vi "dut_tx_test.vi"(11 "TV Parameters(DataType)":T1 {"Standard" items=["80211A/G/J/P OFDM", "80211B/G DSSS", "80211G DSSSOFDM", "80211N MIMOOFDM", "80211AC MIMOOFDM"]; "OFDM Data Rate (Mbps)" items=["6", "9", "12", "18", "24", "36", "48", "54"]; "80211n PLCP Frame Format" items=["Mixed Format", "Greenfield Format"]; "FEC Coding Type" items=["BCC", "LDPC"]; "DSSS Data Rate (Mbps)" items=["1", "2", "5.5 CCK", "5.5 PBCC", "11 CCK", "11 PBCC", "22", "33"]}) -> (3 "Command Sent":string)   [LabVIEW 2011]
uses:
  TV/RW/Includes/WLAN - TV - RW - INC - TV_DataType_Cluster.ctl
  Controls/Transmit Config.ctl
  Controls/Data Rates.ctl
  Controls/Inter Frame Spacing modes.ctl
  Controls/Parameter.ctl
panel:
  in  "OFDM Data Rate (Mbps)":i32(ring) items=["6", "9", "12", "18", "24", "36", "48", "54"]
  out "Messages Logged":string[](array[string])
  in  "error in (no error)":errorcluster
  out "error out":errorcluster
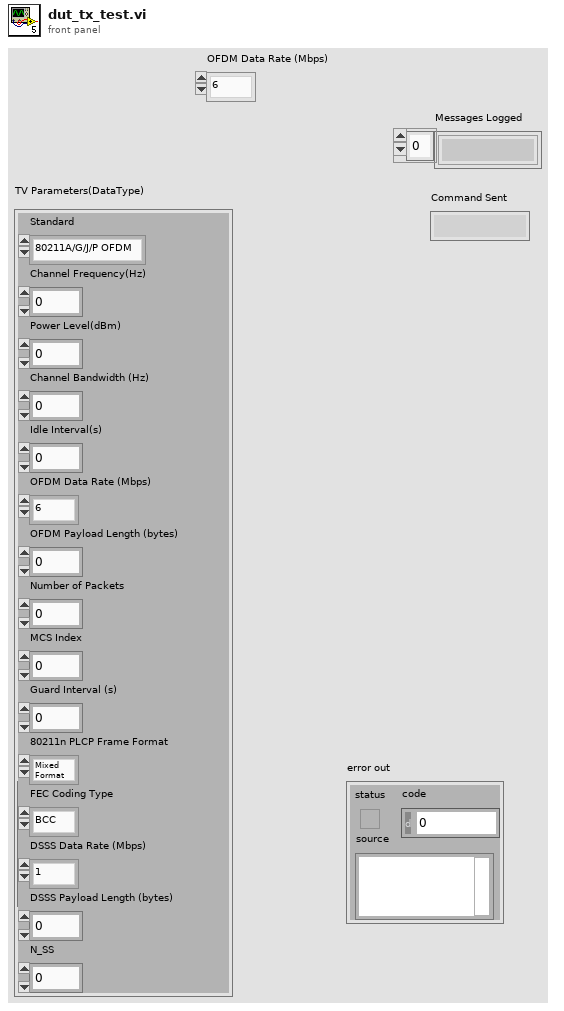
[diagram p1: front panel]
types:
  T1 = typedef "WLAN - TV - RW - INC - TV_DataType_Cluster.ctl" = cluster{"Standard":i32, "Channel Frequency(Hz)":dbl, "Power Level(dBm)":dbl, "Channel Bandwidth (Hz)":dbl, "Idle Interval(s)":dbl, "OFDM Data Rate (Mbps)":i32, "OFDM Payload Length (bytes)":i32, "Number of Packets":i32, "MCS Index":i32, "Guard Interval (s)":dbl, "80211n PLCP Frame Format":i32, "FEC Coding Type":i32, "DSSS Data Rate (Mbps)":i32, "DSSS Payload Length (bytes)":i32, "N_SS":i32}
  T2 = typedef "Data Rates.ctl" = string
  T3 = typedef "Transmit Config.ctl" = cluster{"Packet Length":u32, "Packet Count":i32, "Data Rate":T2, "Frequency, MHz":u32, "Continuous Frames":bool, "TX Power, dB":dbl}
  T4 = enum16{"none", "combined", "isolated", "iterate-combined ", "iterate-isolated"}
  T5 = typedef "Parameter.ctl" = cluster{"Name":string, "Type":enum16{"decimal", "string", "float", "hex"}}
  T6 = typedef "Inter Frame Spacing modes.ctl" = i16
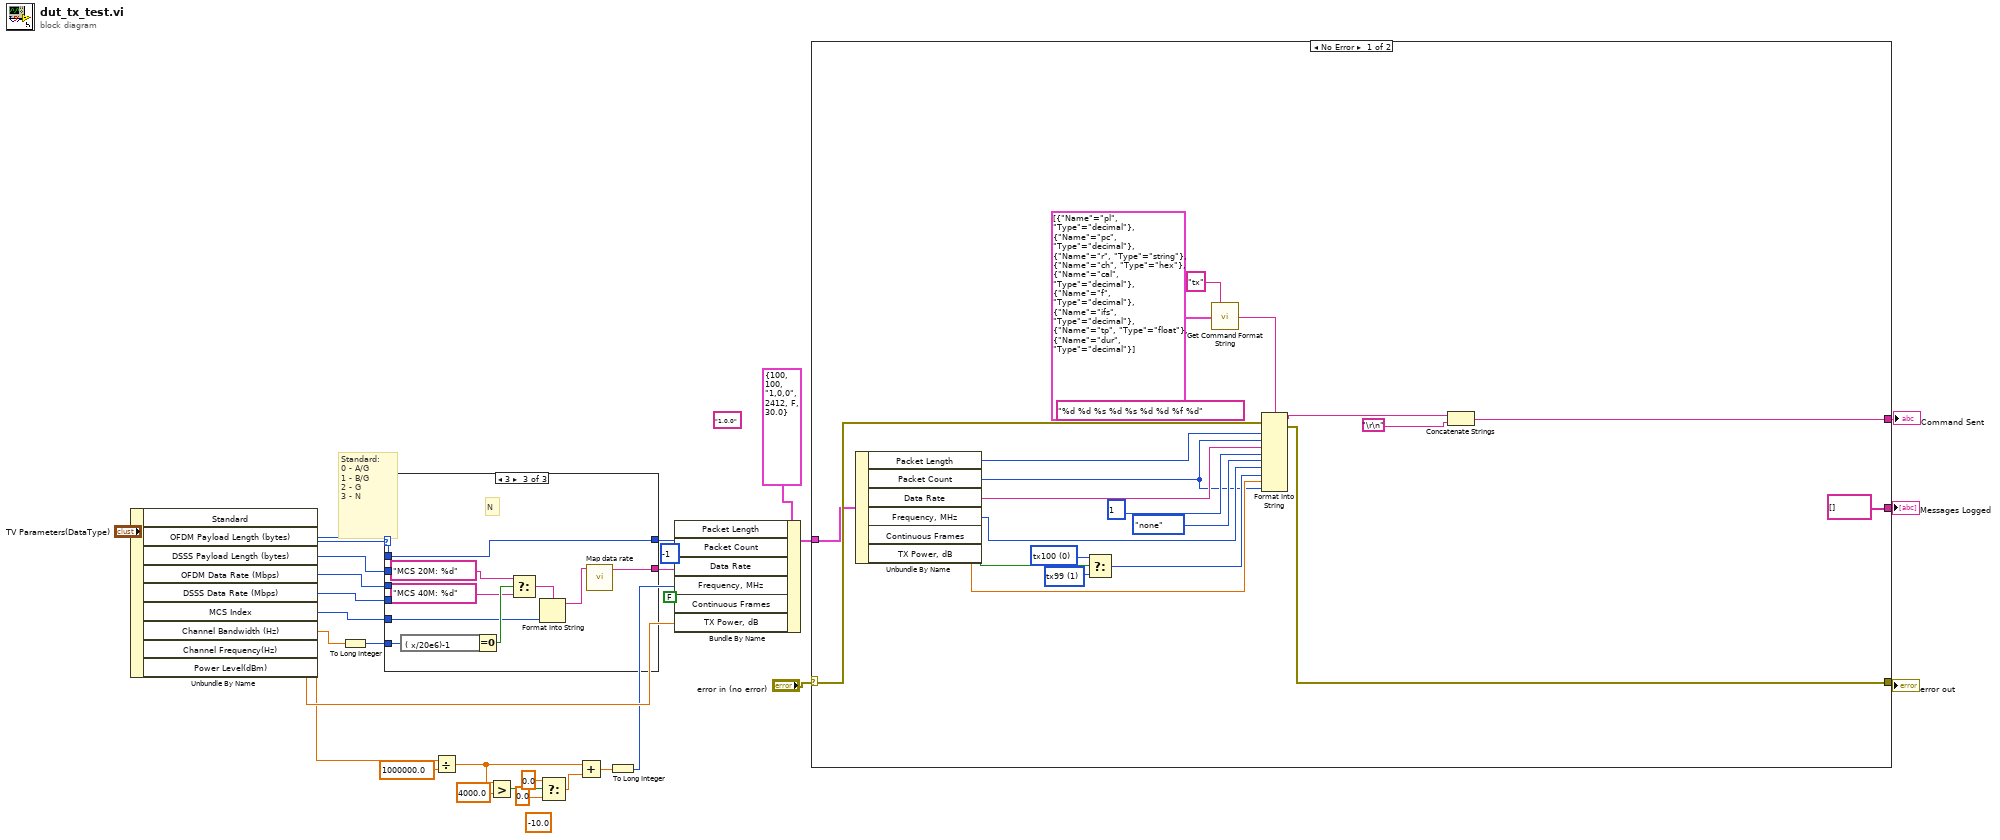
[diagram p0: block diagram]
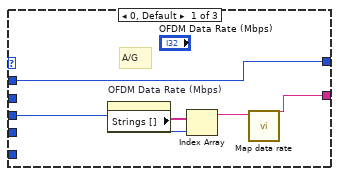
[diagram p2: hidden frame]
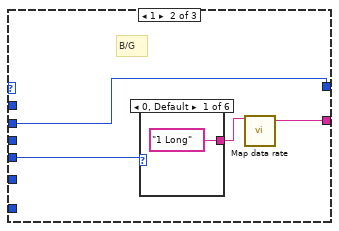
[diagram p3: hidden frame]
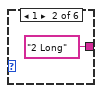
[diagram p4: hidden frame]
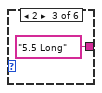
[diagram p5: hidden frame]
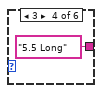
[diagram p6: hidden frame]
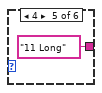
[diagram p7: hidden frame]
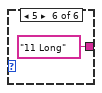
[diagram p8: hidden frame]
diagram:
  (unwired) -10.0 ("t")
  (unwired) T2 "1,0,0" ("Data Rate")
  # "Standard:\n0 - A/G\n1 - B/G\n2 - G\n3 - N"
  n1 = Unbundle By Name("TV Parameters(DataType)") -> ("Standard"=w21:i32, "OFDM Payload Length (bytes)"=w19:i32, "DSSS Payload Length (bytes)"=w18:i32, "OFDM Data Rate (Mbps)"=w17:i32, "DSSS Data Rate (Mbps)"=w15:i32, "MCS Index"=w14:i32, "Channel Bandwidth (Hz)"=w10:dbl, "Channel Frequency(Hz)"=w12:dbl, "Power Level(dBm)"=w16:dbl)
  n2 = To Long Integer(number=w10) -> (32bit integer=w9:i32)
  n3 = case shown="3" w21 {
    tunnel: [w35 w39 w55] -> w20
    tunnel: w19 -> [w35 _ w55]
    tunnel: w18 -> [_ w39 _]
    tunnel: w17 -> [w31 _ _]
    tunnel: w15 -> [_ w38 _]
    tunnel: w14 -> [_ _ w46]
    tunnel: [w34 w37 w54] -> w13
    tunnel: w9 -> [_ _ w47]
    frame 0, Default {
      # "A/G"
      n4 = property on="OFDM Data Rate (Mbps)" class="Ring (strict)"() -> ("Strings []"=w33:string[])  [unwired: 2 in, 2 out]
      n5 = Index Array(array=w33, index=w31) -> (element=w32:string)
      n6 = call "Map data rate.vi"("Data Rate In"=w32) -> ("Data Rate Out"=w34:string)  [unwired: 10 in]
    }
    frame 1 {
      # "B/G"
      n7 = case shown="0, Default" w38 {
        tunnel: ["1 Long" ("Data Rate In") "2 Long" ("Data Rate In") "5.5 Long" ("Data Rate In") "5.5 Long" ("Data Rate In") "11 Long" ("Data Rate In") "11 Long" ("Data Rate In")] -> w36
        frame 0, Default {
        }
        frame 1 {
        }
        frame 2 {
        }
        frame 3 {
        }
        frame 4 {
        }
        frame 5 {
        }
      }
      n8 = call "Map data rate.vi"("Data Rate In"=w36) -> ("Data Rate Out"=w37:string)  [unwired: 10 in]
    }
    frame 3 {
      # "N"
      n9 = expression code="( x/20e6)-1"(w47) -> (w51:i32)
      n10 = Equal To 0?(x=w51) -> (x = 0?=w52:bool)
      n11 = Select(t="MCS 20M: %d" ("format string"), s=w52, f="MCS 40M: %d" ("format string")) -> (s? t:f=w53:string)
      n12 = Format Into String(format string=w53, w46) -> (resulting string=w48:string)  [unwired: 2 in, 1 out]
      n13 = call "Map data rate.vi"("Data Rate In"=w48) -> ("Data Rate Out"=w54:string)  [unwired: 10 in]
    }
  }
  n14 = Divide(x=w12, y=1000000.0 ("x")) -> (x/y=w8:dbl)
  n15 = Greater?(x=w8, y=4000.0) -> (0:w6:bool)
  n16 = Select(t=0.0, s=w6, f=0.0) -> (s? t:f=w2:dbl)
  n17 = Add(x=w8, y=w2) -> (x+y=w3:dbl)
  n18 = To Long Integer(number=w3) -> (32bit integer=w1:i32)
  n19 = Bundle By Name(cluster=T3 {"Packet Length"=100, "Packet Count"=100, "Data Rate"="1,0,0", "Frequency, MHz"=2412, "Continuous Frames"=FALSE, "TX Power, dB"=30.0} ("Transmit Config"), "Packet Length"=w20, "Packet Count"=-1, "Data Rate"=w13, "Frequency, MHz"=w1, "Continuous Frames"=FALSE, "TX Power, dB"=w16) -> (w25:T3)
  n20 = case shown="No Error" "error in (no error)" {
    selector: "error in (no error)" -> [w76 w77]
    tunnel: [w56 w77] -> w29
    tunnel: [string[] [] ("Messages Logged") _] -> w28
    tunnel: [w69 _] -> w27
    tunnel: w25 -> [w57 _]
    frame No Error {
      (unwired) "%d %d %s %d %s %d %d %f %d" ("format string")
      w63 = T6 1 items=["Regular"=-1, "tx100"=0, "tx99"=1] ("ART2 Data.Transmit Config.Inter Frame Spacing")
      w64 = T6 0 items=["Regular"=-1, "tx100"=0, "tx99"=1] ("ART2 Data.Transmit Config.Inter Frame Spacing")
      n21 = Unbundle By Name(w57) -> ("Packet Length"=w75:u32, "Packet Count"=w60:i32, "Data Rate"=w67:T2, "Frequency, MHz"=w72:u32, "Continuous Frames"=w62:bool, "TX Power, dB"=w70:dbl)
      n22 = Select(t=w64, s=w62, f=w63) -> (s? t:f=w61:T6)
      n23 = call "Get Command Format String.vi"("Command"="tx", "Parameters"=T5[] [{"Name"="pl", "Type"=enum."decimal"}, {"Name"="pc", "Type"=enum."decimal"}, {"Name"="r", "Type"=enum."string"}, {"Name"="ch", "Type"=enum."hex"}, {"Name"="cal", "Type"=enum."decimal"}, {"Name"="f", "Type"=enum."decimal"}, {"Name"="ifs", "Type"=enum."decimal"}, {"Name"="tp", "Type"=enum."float"}, {"Name"="dur", "Type"=enum."decimal"}]) -> ("Command Format String"=w71:string)  [unwired: 13 in]
      n24 = Format Into String(format string=w71, error in=w76, w75, w60, w67, u32 1 ("Chains"), T4."none" ("input 5"), w72, w61, w70, w60) -> (resulting string=w59:string, error out=w56:errorcluster)  [unwired: 1 in]
      n25 = Concatenate Strings(w59, "\r\n") -> (w69:string)
    }
    frame Error {
    }
  }
  "error out" <- w29
  "Messages Logged" <- w28
  "Command Sent" <- w27
